vi "ScanString.vi"(8 "error in (no error)":errorcluster, 10 "String":string, 11 "U32 D Element in":refnum<class "U32 D Element.lvclass">) -> (0 "error out":errorcluster, 3 "U32 D Element out":refnum<class "U32 D Element.lvclass">)   [LabVIEW 2020, in "D Datagrid Library.lvlib" / "U32 D Element.lvclass"]
uses:
  U32 D Element.lvclass
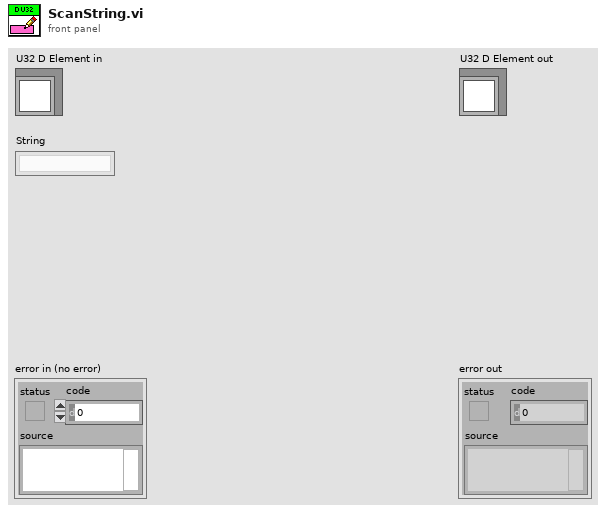
[diagram p1: front panel]
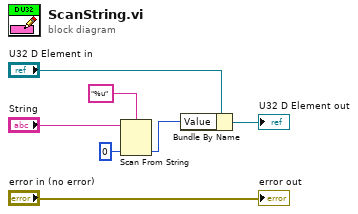
[diagram p0: block diagram]
diagram:
  n1 = Scan From String(format string="%u", input string="String", default 1=u32 0 ("default value 1")) -> (output 1=w6:u32)  [unwired: 2 in, 3 out]
  n2 = Bundle By Name(cluster="U32 D Element in", "Value"=w6) -> (→"U32 D Element out":refnum<class "U32 D Element.lvclass">)
  "error out" <- "error in (no error)"
